vi "Check DMA Blocks Settings.vi"(8 "error in (no error)":errorcluster, 10 "Array in":string[][](array[string]), 11 "DMA Blocks Names In":string[](array[string])) -> (0 "error out":errorcluster, 3 "DMA Blocks Names Out":string[](array[string]))   [LabVIEW 2019, in "RefMem DMA System Explorer.lvlib"]
uses:
  <userlib>/_OpenG.lib/md5/md5.llb/MD5 Message Digest (Binary String)__ogtk.vi
  <userlib>/_OpenG.lib/array/array.llb/Filter 1D Array with Scalar (String)__ogtk.vi
  RefMem DMA System Explorer.lvlib
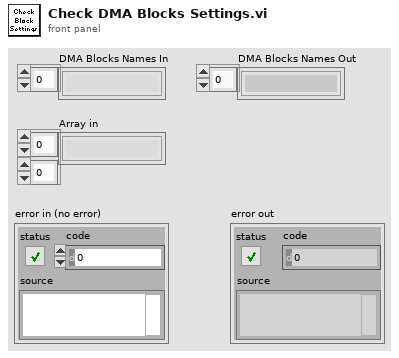
[diagram p1: front panel]
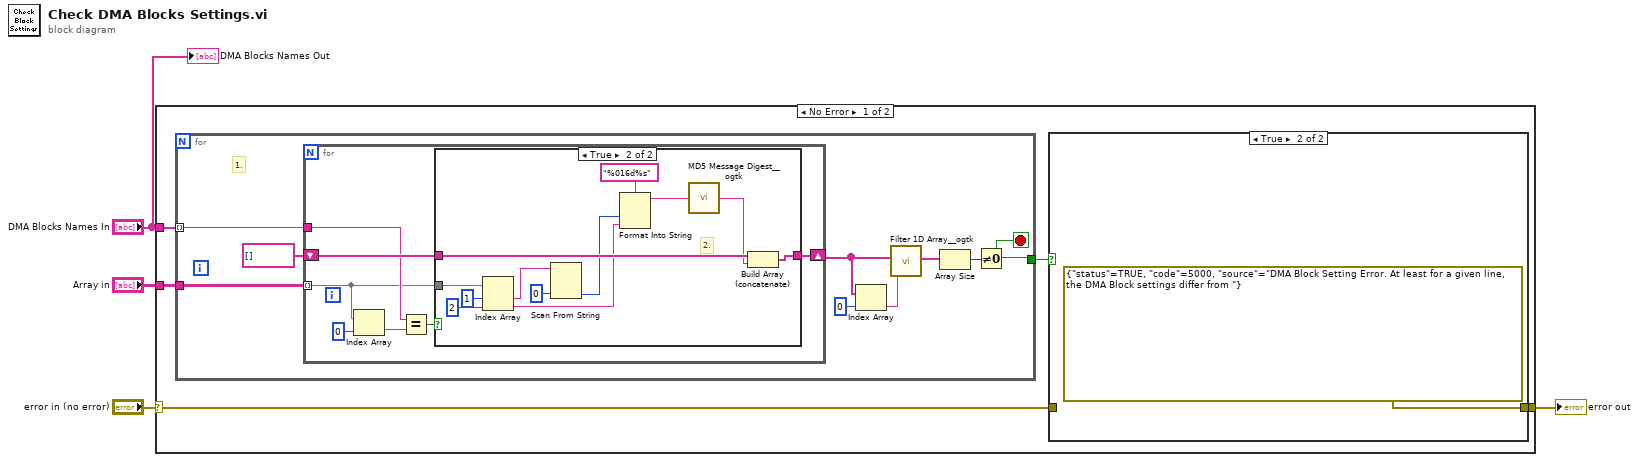
[diagram p0: block diagram]
diagram:
  n1 = case shown="No Error" "error in (no error)" {
    selector: "error in (no error)" -> [w6 w41]
    tunnel: "Array in" -> [w9 _]
    tunnel: "DMA Blocks Names In" -> [w8 _]
    tunnel: [w5 w41] -> w2
    frame No Error {
      n2 = for {
        tunnel: w8 -> [w19] mode=indexing
        tunnel: w9 -> [w20]
        tunnel: [w12] -> w7
        stop <- w12 stop-if-true
        # "1."
        n3 = for {
          shift-right: [w26] -> w17
          shift-left: string[] [] -> [w27]
          tunnel: w20 -> [w21] mode=indexing
          tunnel: w19 -> [w23]
          n4 = Index Array(array=w21, index=0) -> (element=w24:string)
          n5 = Equal?(x=w23, y=w24) -> (x = y?=w22:bool)
          n6 = case shown="True" w22 {
            tunnel: w27 -> [w28 w40]
            tunnel: [w28 w39] -> w26
            tunnel: w21 -> [_ w35]
            frame False {
            }
            frame True {
              # "2."
              n7 = Index Array(array=w35, index #1=1 ("index"), index #2=2 ("index")) -> (element #1=w33:string, element #2=w29:string)
              n8 = Scan From String(input string=w33, default 1=u32 0) -> (output 1=w30:u32)  [unwired: 3 in, 3 out]
              n9 = Format Into String(format string="%016d%s", w30, w29) -> (resulting string=w37:string)  [unwired: 2 in, 1 out]
              n10 = call-poly <userlib>:"MD5 Message Digest__ogtk.vi"("Message"=w37) -> ("MD5 Message Digest"=w36:string)
              n11 = Build Array (concatenate)(w40, w36) -> (w39:string[])
            }
          }
        }
        n12 = Index Array(array=w17, index=0) -> (element=w15:string)
        n13 = call-poly <userlib>:"Filter 1D Array__ogtk.vi"("items to filter"=w15, "array"=w17) -> ("filtered array"=w14:string[])  [unwired: 4 in, 1 out]
        n14 = Array Size(array=w14) -> (size(s)=w13:i32)
        n15 = Not Equal To 0?(x=w13) -> (x != 0?=w12:bool)
      }
      n16 = case shown="True" w7 {
        tunnel: w6 -> [w10 _]
        tunnel: [w10 errorcluster {"status"=TRUE, "code"=5000, "source"="DMA Block Setting Error. At least for a given line, the DMA Block settings differ from "} ("error IO")] -> w5
        frame False {
        }
        frame True {
        }
      }
    }
    frame Error {
    }
  }
  "error out" <- w2
  "DMA Blocks Names Out" <- "DMA Blocks Names In"
